vi "Destroy.vi"(8 "error in (no error)":errorcluster, 11 "Mock Result Observer in":refnum<class "Mock Result Observer.lvclass">) -> (0 "error out":errorcluster, 2 "Remaining Results":i32)   [LabVIEW 2020, in "Mock Result Observer.lvclass"]
uses:
  Mock Result Observer.lvclass
  Mock Result Observer.lvclass/Mock Result Observer.ctl
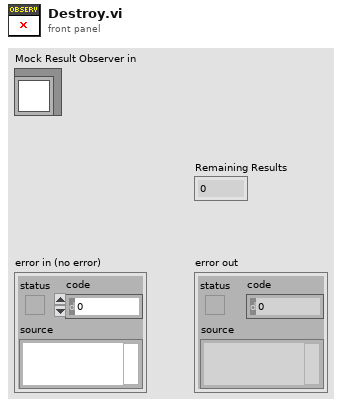
[diagram p1: front panel]
types:
  T1 = typedef "Result.lvlib/Result.ctl" = cluster{"Name":string, "Message":string, "Description":string, "Status":T2, "Result Type":T3, "Execution Time":dbl}
  T2 = typedef "Result.lvlib/Status.ctl" = enum16{"", "Passed", "Failed", "Error", "Skipped", "Setup Error", "Broken", "Teardown Error"}
  T3 = typedef "Result.lvlib/Type.ctl" = enum16{"Method", "Case", "Suite", "Pass", "Fail", "Skip", "Pass if", "Fail if", "Pass if Error", "Fail if Error", "Pass if Equal", "Fail if Equal"}
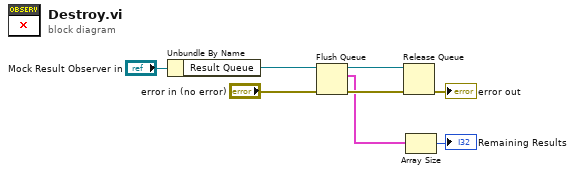
[diagram p0: block diagram]
diagram:
  n1 = Unbundle By Name("Mock Result Observer in") -> ("Result Queue"=w4:refnum<queue>)
  n2 = Flush Queue(queue=w4, error in (no error)="error in (no error)") -> (queue out=w3:refnum<queue>, remaining elements=w2:T1[], error out=w5:errorcluster)
  n3 = Release Queue(queue=w3, error in (no error)=w5) -> (error out=→"error out":errorcluster)  [unwired: 1 in, 2 out]
  n4 = Array Size(array=w2) -> (size(s)=→"Remaining Results":i32)
